vi "Roll_with_complementary_filter.vi"(1 "ax":i32, 2 "az":i32, 3 "% Gyro":dbl=1.0 format="%#_13g", 4 "*roll":dbl) -> (0 "roll":i32)   [LabVIEW 2015]
doc: "roll = atan2(ay,az)*(180/pi)"
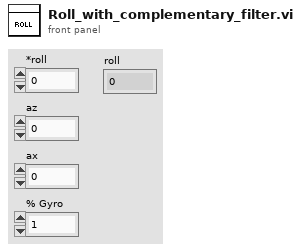
[diagram p1: front panel]
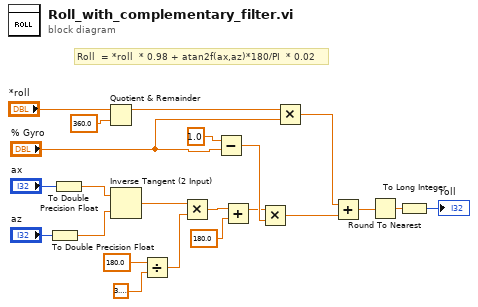
[diagram p0: block diagram]
diagram:
  # "Roll  = *roll  * 0.98 + atan2f(ax,az)*180/PI  * 0.02"
  n1 = To Double Precision Float(number="az") -> (double precision float=w9:dbl)
  n2 = To Double Precision Float(number="ax") -> (double precision float=w10:dbl)
  n3 = Quotient & Remainder(x="*roll", y=360.0) -> (x-y*floor(x/y)=w4:dbl)  [unwired: 1 out]
  n4 = Inverse Tangent (2 Input)(1:w9, 2:w10) -> (0:w22:dbl)
  n5 = Divide(x=180.0, y=3.141592653589793) -> (x/y=w19:dbl)
  n6 = Multiply(x=w22, y=w19) -> (x*y=w16:dbl)
  n7 = Subtract(x=1.0, y="% Gyro") -> (x-y=w6:dbl)
  n8 = Add(x=w16, y=180.0) -> (x+y=w2:dbl)
  n9 = Multiply(x=w2, y=w6) -> (x*y=w13:dbl)
  n10 = Multiply(x=w4, y="% Gyro") -> (x*y=w14:dbl)
  n11 = Add(x=w14, y=w13) -> (x+y=w12:dbl)
  n12 = Round To Nearest(number=w12) -> (nearest integer value=w11:dbl)
  n13 = To Long Integer(number=w11) -> (32bit integer=→"roll":i32)
